vi "Rows Pass.vi"(11 "Color Box":u32(colorbox)=6618880) -> (3 "Frames":T1[](array[typedef]))   [LabVIEW 2019, in "LED Matrix Host.lvlib"]
uses:
  LED Matrix Host.lvlib
  Public/Controls/Frame.ctl
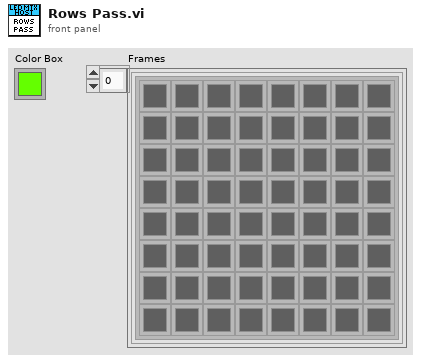
[diagram p1: front panel]
types:
  T1 = typedef "LED Matrix Host.lvlib/Frame.ctl" = cluster{"Matrix":u32[][]}
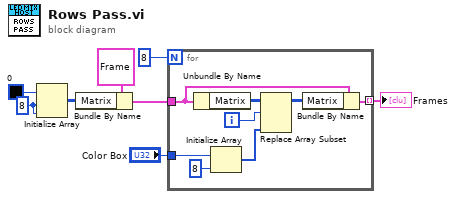
[diagram p0: block diagram]
diagram:
  w2 = 8 ("dimension size")
  n1 = Initialize Array(u32 0 ("Color Box"), w2, w2) -> (w3:u32[][])
  n2 = Bundle By Name(cluster=T1 {"Matrix"=[[0, 0, 0, 0, 0, 0, 0, 0], [16777222, 16777222, 0, 0, 0, 0, 0, 0], [0, 0, 0, 0, 0, 0, 0, 0], [0, 0, 0, 0, 0, 0, 0, 0], [0, 0, 0, 0, 0, 0, 0, 0], [0, 0, 0, 0, 0, 0, 0, 0], [0, 0, 0, 0, 0, 0, 0, 0], [16777222, 0, 0, 0, 0, 0, 0, 16777222]]} ("Matrix"), "Matrix"=w3) -> (w1:T1)
  n3 = for {
    N: 8 -> [_]
    tunnel: w1 -> [w16]
    tunnel: "Color Box" -> [w12]
    tunnel: [w15] -> w7 mode=indexing
    i -> [w9]
    n4 = Unbundle By Name(w16) -> ("Matrix"=w14:u32[][])
    n5 = Initialize Array(w12, 8 ("dimension size")) -> (w10:u32[])
    n6 = Replace Array Subset(array=w14, new element=w10, index (row)=w9) -> (w13:u32[][])  [unwired: 1 in]
    n7 = Bundle By Name(cluster=w16, "Matrix"=w13) -> (w15:T1)
  }
  "Frames" <- w7
